vi "tx_proj.vi"() -> ()   [LabVIEW 2023]
uses:
  <vilib>/addons/Modulation/Analog/support/mod_Set Error Source.vi
  <vilib>/addons/Modulation/Digital/Support/Common/Validators/mod_Generate Filter Coefficients Validate.vi
  <vilib>/addons/Modulation/Digital/General/subVIs/mod_Generate Filter Coefficients.vi
  <vilib>/addons/Modulation/Digital/General/MT Generate QAM System Parameters(M).vi
  <instrlib>/niUSRP/niUSRP Write Tx Data (CDB).vi
  <vilib>/addons/Modulation/niDMT.lvlib
panel:
  out "path out":path
  out "size(s)":i32
  in  "stop":bool
  out "error out":errorcluster
  in  "reset? (T)":bool=TRUE
  in  "active antenna":string
  in  "gain":dbl format="%#_6f"
  in  "carrier frequency":dbl=100000.0 format="%#_6p"
  in  "IQ rate":dbl=100000.0 format="%#_6p"
  in  "error in (no error)":errorcluster
  in  "USRP IP Address":refnum<k15>
  in  "samples per symbol (16)":i32=16
  in  "filter parameter":dbl=0.5 format="%.2f"
  in  "matched samples per symbol (16)":i32=16
  in  "pulse shaping samples per symbol (16)":i32=16
  in  "M-QAM (16)":i32=16
  out "Constellation":T1(graph)
  out "constellation graph":T1(array[cluster]) {"oversampled data" format="%.2f"; "constellation" format="%.2f"}
  in  "pulse shaping filter (none)":T2(ring)
  out "Input":waveform(dbl)(graph)
  in  "path":path
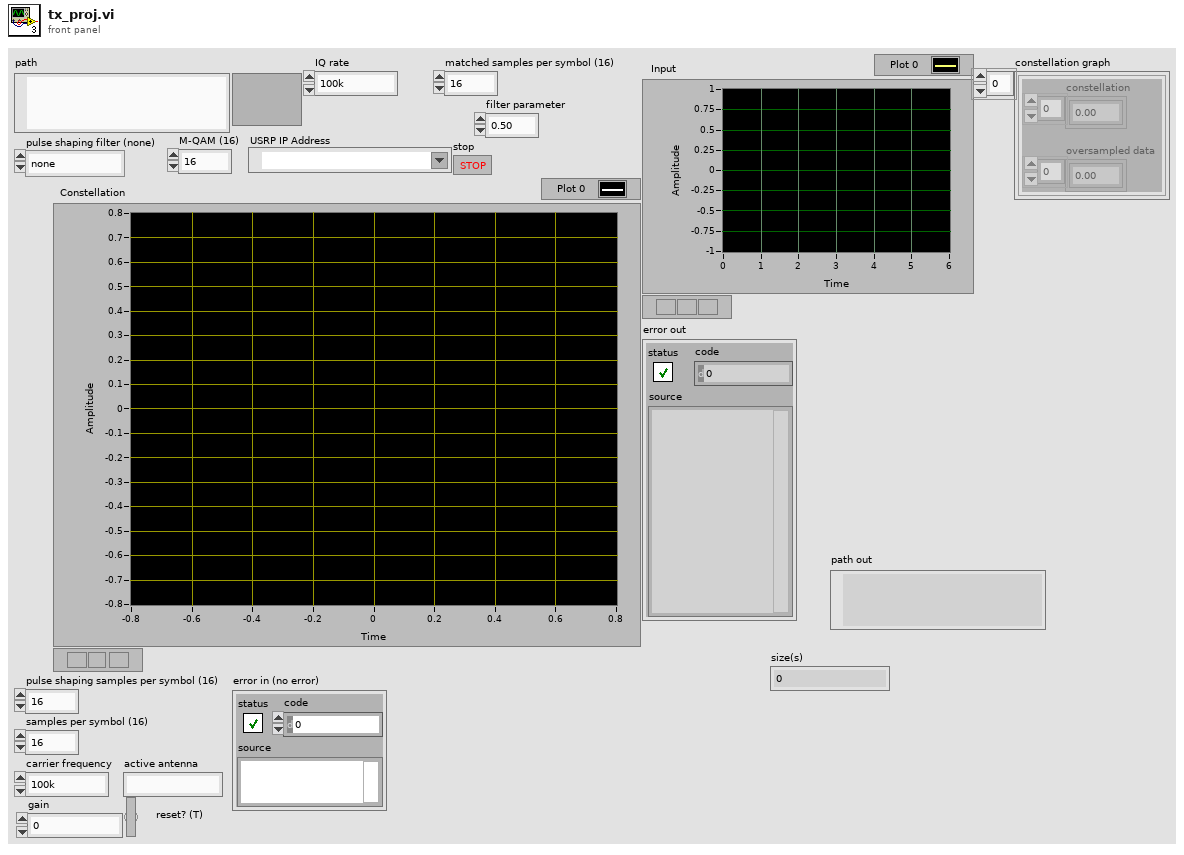
[diagram p1: front panel]
types:
  T1 = cluster{"constellation":dbl[], "oversampled data":dbl[]}[]
  T2 = enum16{"none", "Raised Cosine", "Root Raised Cos", "Gaussian"}
  T3 = enum16{"FSK", "PSK", "QAM", "MSK", "PAM", "ASK", "CPM"}
  T4 = cluster{"samples per symbol (16)":i32, "symbol map":cdb[]}
  T5 = typedef "niAMT.lvlib/Complex Data Waveform.ctl" = cluster{"t0":dbl, "dt":dbl, "Y":cdb[]}
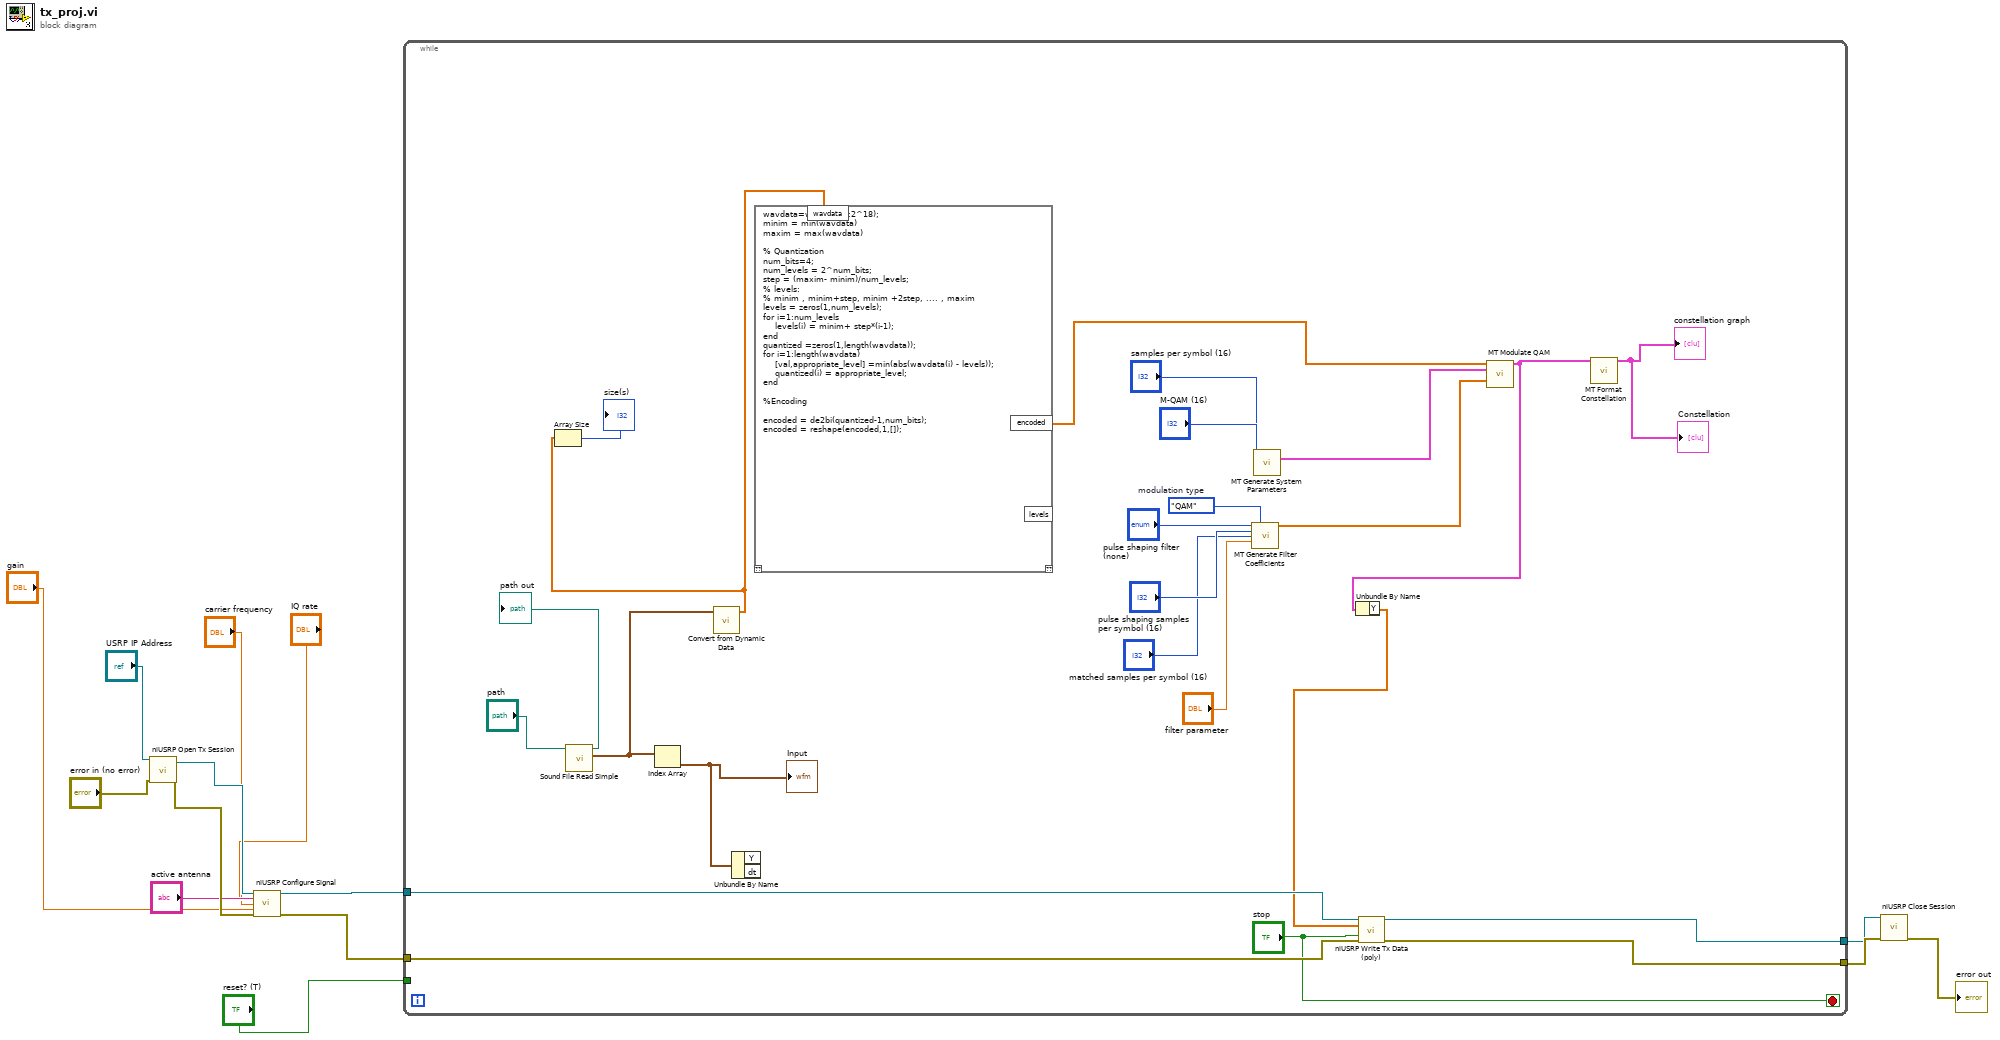
[diagram p0: block diagram]
diagram:
  n1 = call <instrlib>:"niUSRP Open Tx Session.vi"("device names"="USRP IP Address", "error in (no error)"="error in (no error)") -> ("session handle out"=w14:refnum<k15>, "error out"=w13:errorcluster)  [unwired: 12 in]
  n2 = call <instrlib>:"niUSRP Configure Signal.vi"("session handle"=w14, "IQ rate"="IQ rate", "carrier frequency"="carrier frequency", "gain"="gain", "error in (no error)"=w13, "active antenna"="active antenna") -> ("session handle out"=w3:refnum<k15>, "error out"=w2:errorcluster)  [unwired: 5 in, 3 out]
  n3 = while {
    tunnel: [w25] -> w5
    tunnel: [w24] -> w4
    tunnel: w3 -> [w23]
    tunnel: w2 -> [w22]
    tunnel: "reset? (T)" -> [_]
    stop <- "stop" stop-if-true
    w37 = T3."QAM"  # modulation type
    n4 = call <vilib>:"Sound File Read Simple.vi"("path"="path") -> ("data"=w28:waveform(dbl)[], "path out"=→"path out":path)  [unwired: 7 in, 2 out]
    n5 = Index Array "Index Array"(array=w28) -> (element=w29:waveform(dbl))  [unwired: 1 in]
    "Input" <- w29
    n6 = call "Convert from Dynamic Data"("Dynamic Data Type"=w28) -> ("Array"=w17:dbl[])  [unwired: 3 in]
    n7 = Array Size(array=w17) -> (size(s)=→"size(s)":i32)
    n8 = Unbundle By Name(w29) -> ()  [unwired: 2 out]
    n9 = script code="wavdata=wavdata(1:2^18);\nminim = min(wavdata)\nmaxim = max(wavdata)\n\n% Quantization\nnum_bits=4;\nnum_levels = 2^num_bits;\nstep = (maxim- minim)/num_levels;\n% levels:\n% minim , minim+step, minim +2step, .... , maxim\nlevels = zeros(1,num_levels);\nfor i=1:num_levels\n    levels(i) = minim+ step*(i-1);\nend\nquantized =zeros(1,length(wavdata));\nfor i=1:length(wavdata)\n    [val,appropriate_level] =min(abs(wavdata(i) - levels));\n    quantized(i) = appropriate_level;\nend\n\n%Encoding\n\nencoded = de2bi(quantized-1,num_bits);\nencoded = reshape(encoded,1,[]);"("wavdata"=w17) -> ("encoded"=w19:dbl[])  [unwired: 1 in, 2 out]
    n10 = call <vilib>:"MT Generate Filter Coefficients.vi"("pulse shaping filter (none)"="pulse shaping filter (none)", "modulation type"=w37, "pulse shaping samples per symbol (16)"="pulse shaping samples per symbol (16)", "matched samples per symbol (16)"="matched samples per symbol (16)", "filter parameter"="filter parameter") -> ("pulse shaping filter coefficients"=w26:dbl[])  [unwired: 8 in, 2 out]
    n11 = call-poly <vilib>:"MT Generate System Parameters.vi"("samples per symbol (16)"="samples per symbol (16)", "M-QAM (16)"="M-QAM (16)") -> ("QAM system parameters"=w27:T4)  [unwired: 11 in, 2 out]
    n12 = call <vilib>:"MT Modulate QAM.vi"("input bit stream"=w19, "QAM system parameters"=w27, "pulse shaping filter coefficients"=w26) -> ("output complex waveform"=w21:T5)  [unwired: 10 in, 2 out]
    n13 = Unbundle By Name "Unbundle By Name"(w21) -> ("Y"=w20:cdb[])
    n14 = call-poly <instrlib>:"niUSRP Write Tx Data (poly).vi"("session handle"=w23, "data"=w20, "end of data?"="stop", "error in (no error)"=w22) -> ("session handle out"=w24:refnum<k15>, "error out"=w25:errorcluster)  [unwired: 10 in]
    n15 = call <vilib>:"MT Format Constellation.vi"("waveform"=w21) -> ("constellation graph"=→"constellation graph" →"Constellation":T1)  [unwired: 13 in, 1 out]
  }
  n16 = call <instrlib>:"niUSRP Close Session.vi"("session handle"=w4, "error in (no error)"=w5) -> ("error out"=→"error out":errorcluster)  [unwired: 13 in]
